vi "DriverStationGetData.vi"   [LabVIEW 2020]
doc: "This VI recieves data from the FRC 4265 Dashboard continuously, in all robot modes. These may include safety overrides, calibration commands, and configuration parameters. However this VI should never include standard driver or manipulator commands."
uses:
  f2972b46-d919-4210-bfdf-d3cf9c7f3ddc.vi
  GlobalDriverStationData.vi
  <vilib>/Rock Robotics/Network Tables/NT Read Number.vi
  <vilib>/Rock Robotics/Network Tables/NT Read Boolean.vi
  GlobalDrivebase.vi
  GlobalPoseAndTargeting.vi
  <vilib>/Rock Robotics/Network Tables/NT Read Numeric Array.vi
  GlobalDriverStationCommands.vi
  GRNF_Joystick.vi
  <vilib>/Rock Robotics/Network Tables/NT Read String.vi
  <vilib>/Utility/xml.llb/Write to XML File(string).vi
  GlobalActuators.vi
  <vilib>/Rock Robotics/Network Tables/NT Read Integer Array.vi
  <vilib>/Rock Robotics/Network Tables/NT Read Boolean Array.vi
types:
  T1 = enum16{"Center", "North", "NorthWest", "West", "SouthWest", "South", "SouthEast", "East", "NorthEast"}
  T2 = enum16{"Off", "Toggle", "D_LT", "D_RT", "D_LB", "D_RB", "D_Y", "D_X", "D_A", "D_B", "M_LT", "M_RT", "M_LB", "M_RB", "M_Y", "M_X", "M_A", "M_B"}
  T3 = enum16{"Off", "Slider", "D_LT", "D_RT", "D_LB", "D_RB", "D_Y", "D_X", "D_A", "D_B", "M_LJoystick_X", "M_LJoystick_Y", "M_RJoystick_X", "M_RJoystick_Y", "M_LT", "M_RT", "M_LB", "M_RB", "M_Y", "M_X", "M_A", "M_B"}
  T4 = typedef "WPI_JoystickDevRef.ctl" = cluster{"Device":T5}
  T5 = typedef "WPI_JoystickDeviceEnum.ctl" = enum16{"USB 0", "USB 1", "USB 2", "USB 3", "USB 4", "USB 5"}
  T6 = typedef "WPI_DriverStationAllianceInfo.ctl" = enum16{"Red", "Blue", "Invalid"}
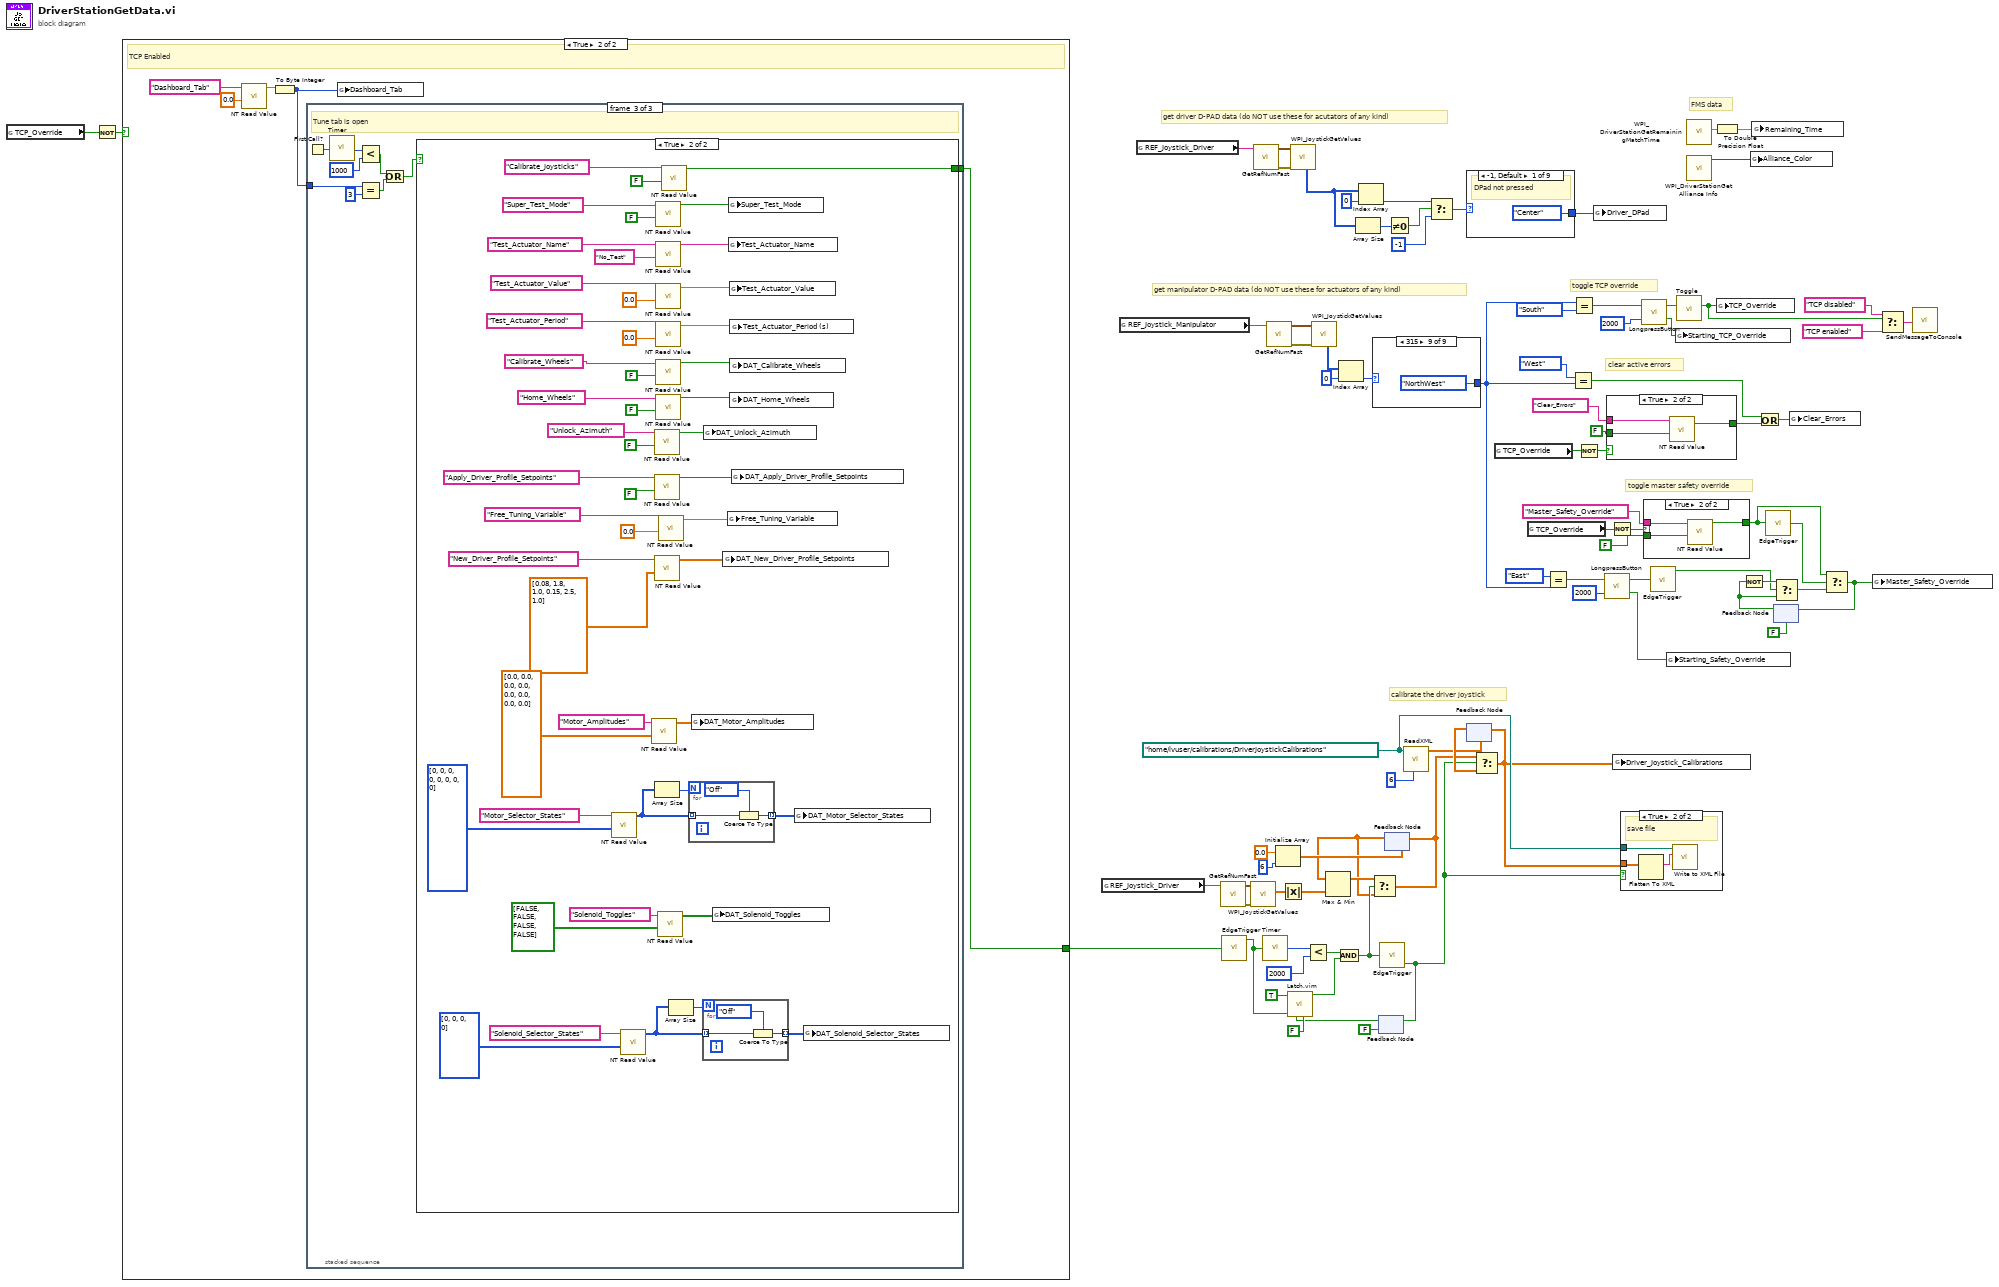
[diagram p0: block diagram]
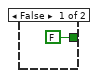
[diagram p2: hidden frame]
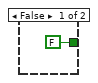
[diagram p3: hidden frame]
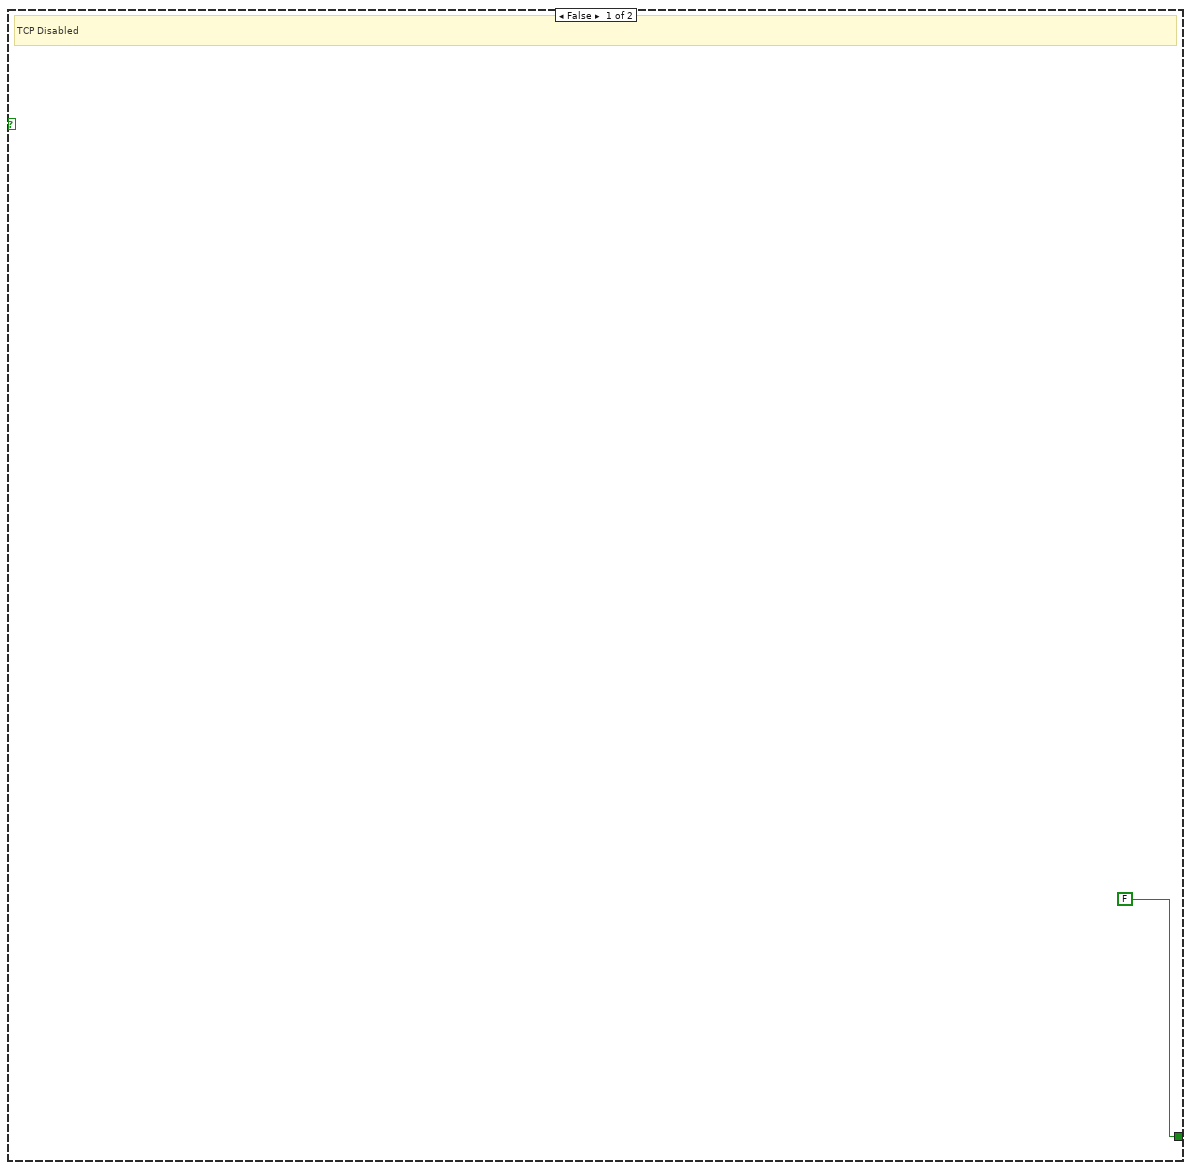
[diagram p4: hidden frame]
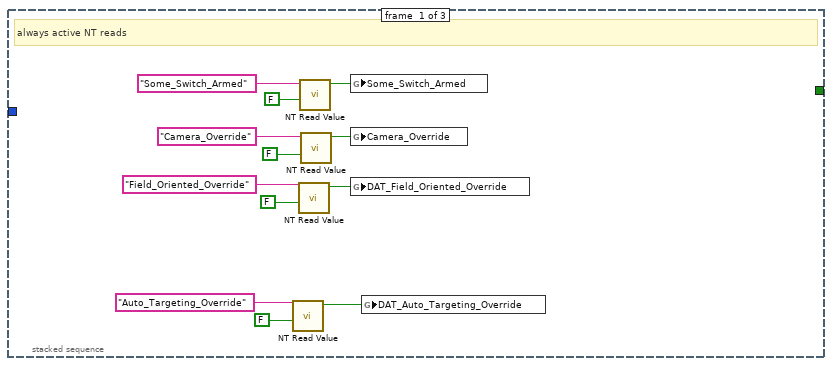
[diagram p5: hidden frame]
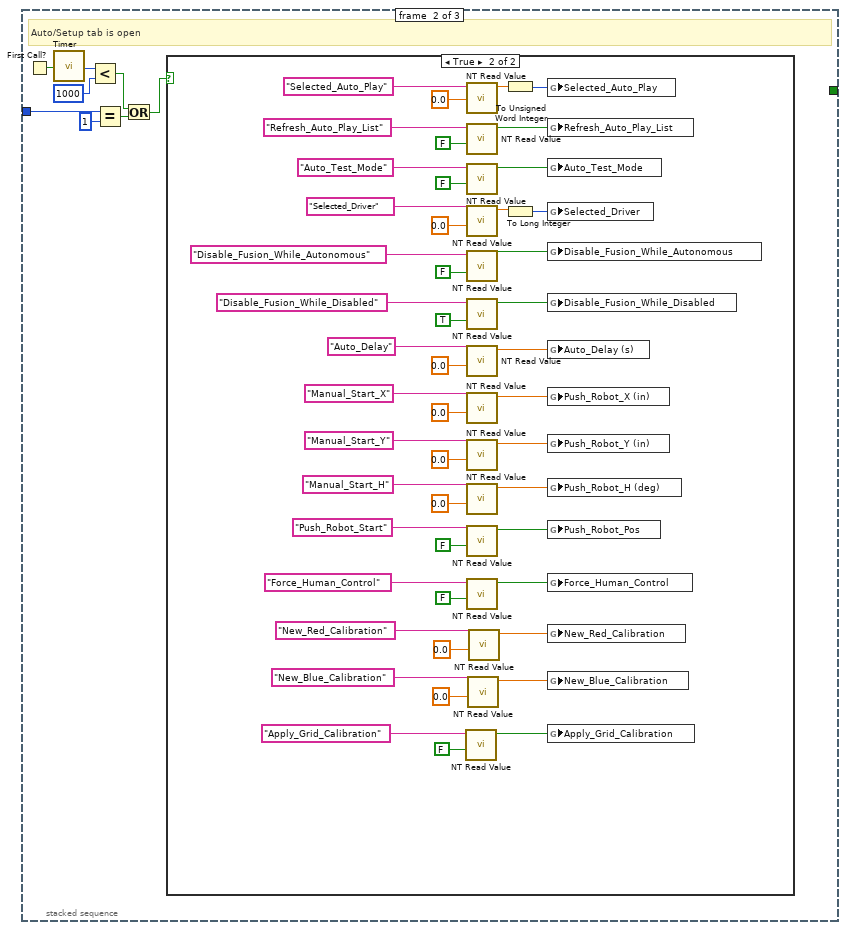
[diagram p6: hidden frame]
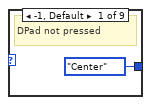
[diagram p9: hidden frame]
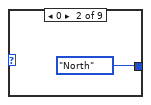
[diagram p10: hidden frame]
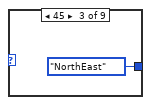
[diagram p11: hidden frame]
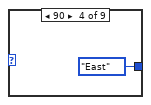
[diagram p12: hidden frame]
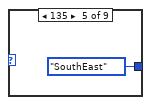
[diagram p13: hidden frame]
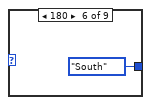
[diagram p14: hidden frame]
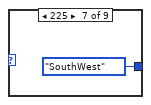
[diagram p15: hidden frame]
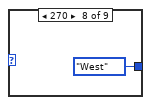
[diagram p16: hidden frame]
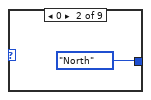
[diagram p17: hidden frame]
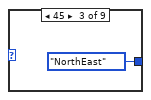
[diagram p18: hidden frame]
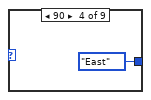
[diagram p19: hidden frame]
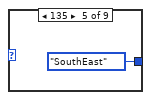
[diagram p20: hidden frame]
diagram:
  w82 = path "/home/lvuser/calibrations/DriverJoystickCalibrations" ("path")
  # "toggle master safety override"
  # "clear active errors"
  # "toggle TCP override"
  # "FMS data"
  # "get manipulator D-PAD data (do NOT use these for actuators of any kind)"
  # "get driver D-PAD data (do NOT use these for acutators of any kind)"
  # "calibrate the driver joystick"
  n1 = global read "GlobalDriverStationData.vi" "TCP_Override"() -> (w15:bool)
  n2 = Not(x=w15) -> (.not. x?=w14:bool)
  n3 = case shown="True" w14 {
    tunnel: [FALSE ("Boolean") w87] -> w26
    frame False {
      # "TCP Disabled"
    }
    frame True {
      # "TCP Enabled"
      n4 = call-poly <vilib>:"NT Read Value.vi"("default value"=0.0 ("Default Value"), "name"="Dashboard_Tab" ("refnum name")) -> ("value"=w89:dbl)  [unwired: 7 in, 2 out]
      n5 = To Byte Integer(number=w89) -> (8bit integer=w88:i8)
      n6 = stacked-sequence {
        tunnel: w88 -> [_ w111 w165]
        tunnel: [_ _ w163] -> w87
        frame #0 {
          # "always active NT reads"
          n7 = call-poly <vilib>:"NT Read Value.vi"("default value"=FALSE ("Default Value"), "name"="Auto_Targeting_Override" ("refnum name")) -> ("value"=w92:bool)  [unwired: 7 in, 2 out]
          n8 = call-poly <vilib>:"NT Read Value.vi"("default value"=FALSE ("Default Value"), "name"="Field_Oriented_Override" ("refnum name")) -> ("value"=w95:bool)  [unwired: 7 in, 2 out]
          n9 = call-poly <vilib>:"NT Read Value.vi"("default value"=FALSE ("Default Value"), "name"="Some_Switch_Armed" ("refnum name")) -> ("value"=w103:bool)  [unwired: 7 in, 2 out]
          n10 = call-poly <vilib>:"NT Read Value.vi"("default value"=FALSE ("Default Value"), "name"="Camera_Override" ("refnum name")) -> ("value"=w100:bool)  [unwired: 7 in, 2 out]
          n11 = global write "GlobalDriverStationData.vi" "Some_Switch_Armed"(w103) -> ()
          n12 = global write "GlobalDriverStationData.vi" "Camera_Override"(w100) -> ()
          n13 = global write "GlobalDrivebase.vi" "DAT_Field_Oriented_Override"(w95) -> ()
          n14 = global write "GlobalDrivebase.vi" "DAT_Auto_Targeting_Override"(w92) -> ()
        }
        frame #1 {
          # "Auto/Setup tab is open"
          n15 = First Call?() -> (First Call?: T/F=w109:bool)
          n16 = call "Timer.vi"("Reset Timer"=w109) -> ("Time (ms)"=w108:u32)
          n17 = Less?(x=w108, y=u32 1000 ("Time threshold (ms)")) -> (x < y?=w106:bool)
          n18 = Equal?(x=w111, y=i8 1) -> (x = y?=w107:bool)
          n19 = Or(x=w106, y=w107) -> (x .or. y?=w105:bool)
          n20 = case shown="True" w105 {
            frame False {
            }
            frame True {
              n21 = call-poly <vilib>:"NT Read Value.vi"("default value"=FALSE ("Default Value"), "name"="Apply_Grid_Calibration" ("refnum name")) -> ("value"=w112:bool)  [unwired: 7 in, 2 out]
              n22 = call-poly <vilib>:"NT Read Value.vi"("default value"=0.0 ("Default Value"), "name"="Selected_Auto_Play" ("refnum name")) -> ("value"=w147:dbl)  [unwired: 7 in, 2 out]
              n23 = call-poly <vilib>:"NT Read Value.vi"("default value"=FALSE ("Default Value"), "name"="Refresh_Auto_Play_List" ("refnum name")) -> ("value"=w146:bool)  [unwired: 7 in, 2 out]
              n24 = call-poly <vilib>:"NT Read Value.vi"("default value"=FALSE ("Default Value"), "name"="Auto_Test_Mode" ("refnum name")) -> ("value"=w158:bool)  [unwired: 7 in, 2 out]
              n25 = call-poly <vilib>:"NT Read Value.vi"("default value"=0.0 ("Default Value"), "name"="Selected_Driver" ("refnum name")) -> ("value"=w149:dbl)  [unwired: 7 in, 2 out]
              n26 = call-poly <vilib>:"NT Read Value.vi"("default value"=FALSE ("Default Value"), "name"="Disable_Fusion_While_Autonomous" ("refnum name")) -> ("value"=w152:bool)  [unwired: 7 in, 2 out]
              n27 = call-poly <vilib>:"NT Read Value.vi"("default value"=TRUE ("Default Value"), "name"="Disable_Fusion_While_Disabled" ("refnum name")) -> ("value"=w153:bool)  [unwired: 7 in, 2 out]
              n28 = call-poly <vilib>:"NT Read Value.vi"("default value"=0.0 ("Default Value"), "name"="Auto_Delay" ("refnum name")) -> ("value"=w151:dbl)  [unwired: 7 in, 2 out]
              n29 = call-poly <vilib>:"NT Read Value.vi"("default value"=0.0 ("Default Value"), "name"="Manual_Start_X" ("refnum name")) -> ("value"=w154:dbl)  [unwired: 7 in, 2 out]
              n30 = call-poly <vilib>:"NT Read Value.vi"("default value"=0.0 ("Default Value"), "name"="Manual_Start_Y" ("refnum name")) -> ("value"=w155:dbl)  [unwired: 7 in, 2 out]
              n31 = call-poly <vilib>:"NT Read Value.vi"("default value"=0.0 ("Default Value"), "name"="Manual_Start_H" ("refnum name")) -> ("value"=w156:dbl)  [unwired: 7 in, 2 out]
              n32 = call-poly <vilib>:"NT Read Value.vi"("default value"=FALSE ("Default Value"), "name"="Push_Robot_Start" ("refnum name")) -> ("value"=w157:bool)  [unwired: 7 in, 2 out]
              n33 = call-poly <vilib>:"NT Read Value.vi"("default value"=FALSE ("Default Value"), "name"="Force_Human_Control" ("refnum name")) -> ("value"=w123:bool)  [unwired: 7 in, 2 out]
              n34 = call-poly <vilib>:"NT Read Value.vi"("default value"=0.0 ("Default Value"), "name"="New_Blue_Calibration" ("refnum name")) -> ("value"=w115:dbl)  [unwired: 7 in, 2 out]
              n35 = call-poly <vilib>:"NT Read Value.vi"("default value"=0.0 ("Default Value"), "name"="New_Red_Calibration" ("refnum name")) -> ("value"=w118:dbl)  [unwired: 7 in, 2 out]
              n36 = To Unsigned Word Integer(number=w147) -> (unsigned 16bit integer=w148:u16)
              n37 = To Long Integer(number=w149) -> (32bit integer=w150:i32)
              n38 = global write "GlobalDriverStationData.vi" "Selected_Auto_Play"(w148) -> ()
              n39 = global write "GlobalDriverStationData.vi" "Refresh_Auto_Play_List"(w146) -> ()
              n40 = global write "GlobalDriverStationData.vi" "Auto_Test_Mode"(w158) -> ()
              n41 = global write "GlobalDriverStationData.vi" "Selected_Driver"(w150) -> ()
              n42 = global write "GlobalDriverStationData.vi" "Disable_Fusion_While_Autonomous"(w152) -> ()
              n43 = global write "GlobalDriverStationData.vi" "Disable_Fusion_While_Disabled"(w153) -> ()
              n44 = global write "GlobalDriverStationData.vi" "Auto_Delay (s)"(w151) -> ()
              n45 = global write "GlobalPoseAndTargeting.vi" "Push_Robot_X (in)"(w154) -> ()
              n46 = global write "GlobalPoseAndTargeting.vi" "Push_Robot_Y (in)"(w155) -> ()
              n47 = global write "GlobalPoseAndTargeting.vi" "Push_Robot_H (deg)"(w156) -> ()
              n48 = global write "GlobalPoseAndTargeting.vi" "Push_Robot_Pos"(w157) -> ()
              n49 = global write "GlobalDriverStationData.vi" "Force_Human_Control"(w123) -> ()
              n50 = global write "GlobalPoseAndTargeting.vi" "New_Red_Calibration"(w118) -> ()
              n51 = global write "GlobalPoseAndTargeting.vi" "New_Blue_Calibration"(w115) -> ()
              n52 = global write "GlobalPoseAndTargeting.vi" "Apply_Grid_Calibration"(w112) -> ()
            }
          }
        }
        frame #2 {
          # "Tune tab is open"
          n53 = First Call?() -> (First Call?: T/F=w162:bool)
          n54 = call "Timer.vi"("Reset Timer"=w162) -> ("Time (ms)"=w161:u32)
          n55 = Less?(x=w161, y=u32 1000 ("Time threshold (ms)")) -> (x < y?=w159:bool)
          n56 = Equal?(x=w165, y=i8 3) -> (x = y?=w167:bool)
          n57 = Or(x=w159, y=w167) -> (x .or. y?=w164:bool)
          n58 = case shown="True" w164 {
            tunnel: [_ w191] -> w163
            frame False {
            }
            frame True {
              n59 = call-poly <vilib>:"NT Read Value.vi"("default value"=i64[] [0, 0, 0, 0, 0, 0, 0, 0] ("DAT_Motor_Selector_States"), "name"="Motor_Selector_States") -> ("value"=w177:i64[])  [unwired: 7 in, 2 out]
              n60 = call-poly <vilib>:"NT Read Value.vi"("default value"=i64[] [0, 0, 0, 0] ("DAT_Motor_Selector_States"), "name"="Solenoid_Selector_States") -> ("value"=w168:i64[])  [unwired: 7 in, 2 out]
              n61 = call-poly <vilib>:"NT Read Value.vi"("default value"=dbl[] [0.0, 0.0, 0.0, 0.0, 0.0, 0.0, 0.0, 0.0], "name"="Motor_Amplitudes") -> ("value"=w181:dbl[])  [unwired: 7 in, 2 out]
              n62 = call-poly <vilib>:"NT Read Value.vi"("default value"=dbl[] [0.08, 1.8, 1.0, 0.15, 2.5, 1.0] ("Default Value"), "name"="New_Driver_Profile_Setpoints" ("Name")) -> ("value"=w187:dbl[])  [unwired: 7 in, 2 out]
              n63 = call-poly <vilib>:"NT Read Value.vi"("default value"=FALSE ("Default Value"), "name"="Unlock_Azimuth" ("refnum name")) -> ("value"=w184:bool)  [unwired: 7 in, 2 out]
              n64 = call-poly <vilib>:"NT Read Value.vi"("default value"=FALSE ("Default Value"), "name"="Apply_Driver_Profile_Setpoints" ("Name")) -> ("value"=w188:bool)  [unwired: 7 in, 2 out]
              n65 = Array Size(array=w177) -> (size(s)=w178:i32)
              n66 = call-poly <vilib>:"NT Read Value.vi"("default value"=FALSE ("Default Value"), "name"="Super_Test_Mode" ("refnum name")) -> ("value"=w216:bool)  [unwired: 7 in, 2 out]
              n67 = call-poly <vilib>:"NT Read Value.vi"("default value"="No_Test" ("Default Value"), "name"="Test_Actuator_Name" ("refnum name")) -> ("value"=w211:string)  [unwired: 7 in, 2 out]
              n68 = call-poly <vilib>:"NT Read Value.vi"("default value"=0.0 ("Default Value"), "name"="Test_Actuator_Value" ("refnum name")) -> ("value"=w212:dbl)  [unwired: 7 in, 2 out]
              n69 = call-poly <vilib>:"NT Read Value.vi"("default value"=0.0 ("Default Value"), "name"="Test_Actuator_Period" ("refnum name")) -> ("value"=w213:dbl)  [unwired: 7 in, 2 out]
              n70 = call-poly <vilib>:"NT Read Value.vi"("default value"=FALSE ("Default Value"), "name"="Calibrate_Wheels" ("refnum name")) -> ("value"=w190:bool)  [unwired: 7 in, 2 out]
              n71 = call-poly <vilib>:"NT Read Value.vi"("default value"=FALSE ("Default Value"), "name"="Home_Wheels" ("refnum name")) -> ("value"=w189:bool)  [unwired: 7 in, 2 out]
              n72 = call-poly <vilib>:"NT Read Value.vi"("default value"=bool[] [FALSE, FALSE, FALSE, FALSE] ("DAT_Solenoid_Toggles"), "name"="Solenoid_Toggles") -> ("value"=w173:bool[])  [unwired: 7 in, 2 out]
              n73 = call-poly <vilib>:"NT Read Value.vi"("default value"=0.0 ("Default Value"), "name"="Free_Tuning_Variable" ("refnum name")) -> ("value"=w197:dbl)  [unwired: 7 in, 2 out]
              n74 = call-poly <vilib>:"NT Read Value.vi"("default value"=FALSE ("Default Value"), "name"="Calibrate_Joysticks" ("refnum name")) -> ("value"=w191:bool)  [unwired: 7 in, 2 out]
              n75 = Array Size(array=w168) -> (size(s)=w170:i32)
              n76 = for {
                N: w178 -> [_]
                tunnel: w177 -> [w221] mode=indexing
                tunnel: [w220] -> w176 mode=indexing
                n77 = Coerce To Type(0:w221, 1:T3."Off" ("Motor 1 Button Selector")) -> (2:w220:T3)
              }
              n78 = global write "GlobalActuators.vi" "DAT_Motor_Amplitudes"(w181) -> ()
              n79 = for {
                N: w170 -> [_]
                tunnel: w168 -> [w219] mode=indexing
                tunnel: [w218] -> w169 mode=indexing
                n80 = Coerce To Type(0:w219, 1:T2."Off" ("Solenoid 1 Selector")) -> (2:w218:T2)
              }
              n81 = global write "GlobalDrivebase.vi" "DAT_Unlock_Azimuth"(w184) -> ()
              n82 = global write "GlobalActuators.vi" "DAT_Solenoid_Toggles"(w173) -> ()
              n83 = global write "GlobalDrivebase.vi" "DAT_New_Driver_Profile_Setpoints"(w187) -> ()
              n84 = global write "GlobalDriverStationData.vi" "Free_Tuning_Variable"(w197) -> ()
              n85 = global write "GlobalDriverStationData.vi" "Super_Test_Mode"(w216) -> ()
              n86 = global write "GlobalDriverStationData.vi" "Test_Actuator_Name"(w211) -> ()
              n87 = global write "GlobalDriverStationData.vi" "Test_Actuator_Value"(w212) -> ()
              n88 = global write "GlobalDriverStationData.vi" "Test_Actuator_Period (s)"(w213) -> ()
              n89 = global write "GlobalDrivebase.vi" "DAT_Calibrate_Wheels"(w190) -> ()
              n90 = global write "GlobalDrivebase.vi" "DAT_Home_Wheels"(w189) -> ()
              n91 = global write "GlobalDrivebase.vi" "DAT_Apply_Driver_Profile_Setpoints"(w188) -> ()
              n92 = global write "GlobalActuators.vi" "DAT_Motor_Selector_States"(w176) -> ()
              n93 = global write "GlobalActuators.vi" "DAT_Solenoid_Selector_States"(w169) -> ()
            }
          }
        }
      }
      n94 = global write "GlobalDriverStationData.vi" "Dashboard_Tab"(w88) -> ()
    }
  }
  n95 = global read "GlobalDriverStationCommands.vi" "REF_Joystick_Driver"() -> (w7:string)
  n96 = global read "GlobalDriverStationCommands.vi" "REF_Joystick_Manipulator"() -> (w8:string)
  n97 = global read "GlobalDriverStationCommands.vi" "REF_Joystick_Driver"() -> (w9:string)
  n98 = call-poly "GetRefNumFast.vi"("RefNum Name"=w7) -> ("Error"=w77:errorcluster, "Device Reference"=w78:T4)  [unwired: 5 in]
  n99 = call "EdgeTrigger.vi"("Input Signal"=w26) -> ("Rising Edge Trigger"=w76:bool)  [unwired: 2 out]
  n100 = call <vilib>:"WPI_JoystickGetValues.vi"("error in (no error)"=w77, "JoystickDevRef"=w78) -> ("Axes"=w66:dbl[])  [unwired: 5 in, 4 out]
  n101 = call-poly "GetRefNumFast.vi"("RefNum Name"=w9) -> ("Error"=w56:errorcluster, "Device Reference"=w57:T4)  [unwired: 5 in]
  n102 = call "Timer.vi"("Reset Timer"=w76) -> ("Time (ms)"=w80:u32)
  n103 = call-poly "GetRefNumFast.vi"("RefNum Name"=w8) -> ("Error"=w84:errorcluster, "Device Reference"=w85:T4)  [unwired: 5 in]
  n104 = Initialize Array(0.0 ("element"), 6 ("dimension size")) -> (w59:dbl[])
  n105 = Absolute Value(x=w66) -> (abs(x)=w63:dbl[])
  n106 = call <vilib>:"WPI_JoystickGetValues.vi"("error in (no error)"=w56, "JoystickDevRef"=w57) -> ("POVs"=w6:i16[])  [unwired: 5 in, 4 out]
  n107 = Less?(x=w80, y=u32 2000) -> (x < y?=w73:bool)
  n108 = call <vilib>:"WPI_JoystickGetValues.vi"("error in (no error)"=w84, "JoystickDevRef"=w85) -> ("POVs"=w51:i16[])  [unwired: 5 in, 4 out]
  n109 = Index Array(array=w51, index=0) -> (element=w52:i16)
  n110 = Array Size(array=w6) -> (size(s)=w5:i32)
  n111 = Index Array(array=w6, index=0) -> (element=w4:i16)
  n112 = case shown="315" w52 {
    tunnel: [T1."Center" T1."North" T1."NorthEast" T1."East" T1."SouthEast" T1."South" T1."SouthWest" T1."West" T1."NorthWest"] -> w24
    frame -1, Default {
      # "DPad not pressed"
    }
    frame 0 {
    }
    frame 45 {
    }
    frame 90 {
    }
    frame 135 {
    }
    frame 180 {
    }
    frame 225 {
    }
    frame 270 {
    }
    frame 315 {
    }
  }
  n113 = feedback #1(FALSE ("Falling Edge Trigger")) -> (w70:bool)
  n114 = call "Latch.vim"("Default Value"=FALSE, "Reset"=w70, "Latch Signal"=w76, "Latch Value"=TRUE) -> ("Latched"=w72:bool)  [unwired: 7 in]
  n115 = And(x=w73, y=w72) -> (x .and. y?=w71:bool)
  n116 = call "EdgeTrigger.vi"("Input Signal"=w71) -> ("Falling Edge Trigger"=w68:bool)  [unwired: 2 out]
  n117 = feedback-in #1(w68) -> ()
  n118 = feedback #2(w59) -> (w58:dbl[])
  n119 = Max & Min(x=w58, y=w63) -> (max(x,y)=w65:dbl[])  [unwired: 1 out]
  n120 = Select(t=w65, s=w71, f=w58) -> (s? t:f=w64:dbl[])
  n121 = feedback-in #2(w64) -> ()
  n122 = Not Equal To 0?(x=w5) -> (x != 0?=w3:bool)
  n123 = call "ReadXML.vi"("Default Number of Elements"=6, "File Path (.xml)"=w82) -> ("Data"=w81:dbl[])  [unwired: 8 in, 1 out]
  n124 = Select(t=w4, s=w3, f=i16 -1) -> (s? t:f=w2:i16)
  n125 = case shown="-1, Default" w2 {
    tunnel: [T1."Center" T1."North" T1."NorthEast" T1."East" T1."SouthEast" T1."South" T1."SouthWest" T1."West" T1."NorthWest"] -> w54
    frame -1, Default {
      # "DPad not pressed"
    }
    frame 0 {
    }
    frame 45 {
    }
    frame 90 {
    }
    frame 135 {
    }
    frame 180 {
    }
    frame 225 {
    }
    frame 270 {
    }
    frame 315 {
    }
  }
  n126 = feedback #3(w81) -> (w83:dbl[])
  n127 = Select(t=w64, s=w68, f=w83) -> (s? t:f=w67:dbl[])
  n128 = feedback-in #3(w67) -> ()
  n129 = global read "GlobalDriverStationData.vi" "TCP_Override"() -> (w11:bool)
  n130 = global read "GlobalDriverStationData.vi" "TCP_Override"() -> (w13:bool)
  n131 = Equal?(x=T1."East", y=w24) -> (x = y?=w40:bool)
  n132 = Equal?(x=T1."West", y=w24) -> (x = y?=w42:bool)
  n133 = Equal?(x=w24, y=T1."South") -> (x = y?=w22:bool)
  n134 = Not(x=w11) -> (.not. x?=w10:bool)
  n135 = global write "GlobalDriverStationData.vi" "Driver_DPad"(w54) -> ()
  n136 = call "LongpressButton.vi"("Threshold (ms)"=u32 2000, "Button"=w40) -> ("Starting Press"=w39:bool, "Longpress Button"=w33:bool)
  n137 = case shown="True" w10 {
    tunnel: FALSE ("Default Value") -> [_ w244]
    tunnel: "Clear_Errors" ("refnum name") -> [_ w243]
    tunnel: [FALSE ("Boolean") w242] -> w43
    frame False {
    }
    frame True {
      n138 = call-poly <vilib>:"NT Read Value.vi"("default value"=w244, "name"=w243) -> ("value"=w242:bool)  [unwired: 7 in, 2 out]
    }
  }
  n139 = Not(x=w13) -> (.not. x?=w12:bool)
  n140 = global write "GlobalDriverStationData.vi" "Driver_Joystick_Calibrations"(w67) -> ()
  n141 = case shown="True" w68 {
    tunnel: w82 -> [_ w247]
    tunnel: w67 -> [_ w246]
    frame False {
    }
    frame True {
      # "save file"
      n142 = Flatten To XML(6:w246) -> (2:w245:string)
      n143 = call-poly <vilib>:"Write to XML File.vi"("XML Input"=w245, "XML File Path"=w247) -> ()  [unwired: 7 in, 3 out]
    }
  }
  n144 = call "LongpressButton.vi"("Threshold (ms)"=u32 2000, "Button"=w22) -> ("Starting Press"=w21:bool, "Longpress Button"=w20:bool)
  n145 = case shown="True" w12 {
    tunnel: FALSE ("Default Value") -> [_ w251]
    tunnel: "Master_Safety_Override" ("refnum name") -> [_ w250]
    tunnel: [FALSE ("Boolean") w249] -> w30
    frame False {
    }
    frame True {
      n146 = call-poly <vilib>:"NT Read Value.vi"("default value"=w251, "name"=w250) -> ("value"=w249:bool)  [unwired: 7 in, 2 out]
    }
  }
  n147 = call "EdgeTrigger.vi"("Input Signal"=w33) -> ("Rising Edge Trigger"=w32:bool)  [unwired: 2 out]
  n148 = global write "GlobalDriverStationData.vi" "Starting_Safety_Override"(w39) -> ()
  n149 = global write "GlobalDriverStationData.vi" "Starting_TCP_Override"(w21) -> ()
  n150 = call "Toggle.vi"("Trigger"=w20) -> ("New State"=w18:bool)  [unwired: 1 in]
  n151 = call <vilib>:"WPI_DriverStationGetRemainingMatchTime.vi"() -> ("Match Time(s)"=w50:sgl)  [unwired: 10 in, 1 out]
  n152 = call <vilib>:"WPI_DriverStationGet Alliance Info.vi"() -> ("Alliance"=w48:T6)  [unwired: 6 in, 5 out]
  n153 = To Double Precision Float(number=w50) -> (double precision float=w49:dbl)
  n154 = global write "GlobalDriverStationData.vi" "TCP_Override"(w18) -> ()
  n155 = global write "GlobalDriverStationData.vi" "Alliance_Color"(w48) -> ()
  n156 = global write "GlobalDriverStationData.vi" "Remaining_Time"(w49) -> ()
  n157 = Or(x=w42, y=w43) -> (x .or. y?=w46:bool)
  n158 = call "EdgeTrigger.vi"("Input Signal"=w30) -> ("All Edge Trigger"=w29:bool)  [unwired: 2 out]
  n159 = feedback #4(FALSE ("Initial State")) -> (w35:bool)
  n160 = Not(x=w35) -> (.not. x?=w36:bool)
  n161 = Select(t=w36, s=w32, f=w35) -> (s? t:f=w31:bool)
  n162 = global write "GlobalDriverStationData.vi" "Clear_Errors"(w46) -> ()
  n163 = Select(t=w30, s=w29, f=w31) -> (s? t:f=w28:bool)
  n164 = feedback-in #4(w28) -> ()
  n165 = global write "GlobalDriverStationData.vi" "Master_Safety_Override"(w28) -> ()
  n166 = Select(t="TCP disabled" ("Message String"), s=w18, f="TCP enabled" ("Message String")) -> (s? t:f=w19:string)
  n167 = call "SendMessageToConsole.vi"("Message String"=w19) -> ()  [unwired: 1 in]
